vi "steer_subvi.vi"(11 "Numeric in":fxp<+,32,3>) -> (3 "Numeric out":sgl)   [LabVIEW 2014]
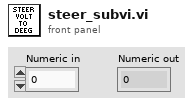
[diagram p1: front panel]
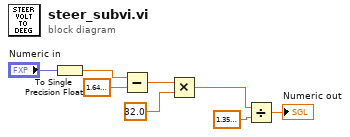
[diagram p0: block diagram]
diagram:
  n1 = To Single Precision Float(number="Numeric in") -> (single precision float=w5:sgl)
  n2 = Subtract(x=w5, y=sgl 1.65) -> (x-y=w3:sgl)
  n3 = Multiply(x=w3, y=sgl 32.0) -> (x*y=w1:sgl)
  n4 = Divide(x=w1, y=sgl 1.35) -> (x/y=→"Numeric out":sgl)
